vi "RT Driver VI.vi"(7 "Operation":T1, 11 "Device Reference in":T2 format="%.0x") -> (0 "Error Code":i32)   [LabVIEW 2021, in "Modbus Master Engine.lvlib"]
uses:
  Modbus Master Engine.lvlib
  <vilib>/NI VeriStand/Custom Device API/Custom Device Item Ref.ctl
  <vilib>/NI VeriStand/Custom Device API/Hardware Interface Driver VI Operation.ctl
  Shared/Device Info.ctl
  Shared/Write Mode.ctl
  Shared/Controls/Interface Type.ctl
  Shared/Controls/Data Model/TCP Settings.ctl
  Shared/Controls/Data Model/Serial Settings.ctl
  SubVIs/Bulk Data Access.ctl
  System Explorer/SubVIs/Modbus Type.ctl
  Shared/Controls/Data Model/Channel.ctl
  <vilib>/NI VeriStand/Custom Device API/Custom Device Channel Type.ctl
  Shared/Controls/Data Model/Mapping.ctl
  Shared/Controls/Data Model/DataType.ctl
  RTStateData.ctl
  <vilib>/NI/NIVS Inline Async API/_VS Inline Async API/VS Inline Async API/VS Inline Async API.lvclass
  <vilib>/NI/NIVS Inline Async API/_VS Inline Async API/VS Inline Async API/VS Inline Async API.lvclass/VS Inline Async API.ctl
  <vilib>/NI/NIVS Inline Async API/_Data Access Engine/Data Access Engine/Data Access Engine.lvclass/Data Access Engine.ctl
  <vilib>/NI/NIVS Inline Async API/_Data Access Engine/Access Type Classes/Write/Write.lvclass/Write.ctl
  <vilib>/NI/NIVS Inline Async API/_Data Access Engine/Access Type Classes/ReadWrite/ReadWrite.lvclass/ReadWrite.ctl
  <vilib>/NI/NIVS Inline Async API/_Data Access Engine/Access Type Classes/Read/Read.lvclass/Read.ctl
  <vilib>/NI/NIVS Inline Async API/_Data Access Engine/Data Access Engine/Methods/Data.Engine.Read Data from HW.vi
  <vilib>/NI/NIVS Inline Async API/_VS Inline Async API/Error Handling Process/SubVIs/Error.GetError.vi
  <vilib>/NI/NIVS Inline Async API/_Data Access Engine/Data Access Engine/Methods/Data.Engine.Write Data to HW.vi
  <vilib>/NI/NIVS Inline Async API/_Data Access Engine/Access Type Classes/ReadWrite/ReadWrite.EngineData.vi
  <vilib>/NI/NIVS Inline Async API/_Data Access Engine/Access Type Classes/Write/Write.EngineData.vi
  <vilib>/NI/NIVS Inline Async API/_Data Access Engine/Access Type Classes/Read/Read.EngineData.vi
  <vilib>/NI VeriStand/Custom Device API/NI VeriStand - Get Channel Value by Data Reference.vi
  <vilib>/NI VeriStand/Custom Device API/NI VeriStand - Set Channel Value by Data Reference.vi
  <vilib>/NI VeriStand/Custom Device API/NI VeriStand - Get Channel Values by Block Data Reference.vi
  Modbus Async.vi
  Shared/Constants.vi
  <vilib>/NI VeriStand/Custom Device API/Get Item Property (Variant).vi
  <vilib>/NI VeriStand/Custom Device API/Global Data Refs.vi
  <vilib>/NI VeriStand/Custom Device API/Custom Device API.lvlib
  Shared/Modbus Master Shared.lvlib
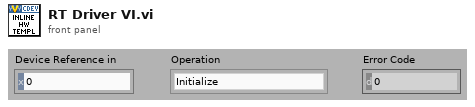
[diagram p1: front panel]
types:
  T1 = typedef "Custom Device API.lvlib/Hardware Interface Driver VI Operation.ctl" = enum16{"Initialize", "Start", "Read Data from HW", "Write Data to HW", "Close"}
  T2 = typedef "Custom Device API.lvlib/Custom Device Item Ref.ctl" = u64
  T3 = typedef "Modbus Master Engine.lvlib/RTStateData.ctl" = cluster{"Async":refnum<class "VS Inline Async API.lvclass">, "Device Info":T4}
  T4 = typedef "Modbus Master Shared.lvlib/Device Info.ctl" = cluster{"Interface Data":cluster{"Name":string, "Unit ID":u8, "Refresh Rate":i32, "Write Rate":i32, "Write Mode":T5, "Interface Type":T6, "TCP Settings":T7, "Serial Settings":T8}, "Modbus Input Groups":T9[], "Modbus Output Groups":T9[], "error in (no error)":errorcluster, "Modbus Input Engine Group Names":string[], "Modbus Output Engine Group Names":string[]}
  T5 = typedef "Modbus Master Shared.lvlib/Write Mode.ctl" = enum16{"Value Change", "Interval"}
  T6 = typedef "Modbus Master Shared.lvlib/Interface Type.ctl" = enum16{"TCP Master", "Serial Master", "TCP Slave", "Serial Slave"}
  T7 = typedef "Modbus Master Shared.lvlib/TCP Settings.ctl" = cluster{"Address":string, "Port":u16, "Timeout":i32}
  T8 = typedef "Modbus Master Shared.lvlib/Serial Settings.ctl" = cluster{"VISA resource name":refnum<visa-resource-name>, "baud rate":u32, "parity (even)":u16, "flow control (none)":u16, "serial type":enum16{"RTU", "ASCII"}, "Wire Mode":i16}
  T9 = typedef "Modbus Master Shared.lvlib/Bulk Data Access.ctl" = cluster{"Modbus Type":T10, "start":u16, "length":u16, "Channel Data":T11[]}
  T10 = typedef "Modbus Master Shared.lvlib/Modbus Type.ctl" = enum16{"Coil", "Discrete Input", "Holding Register", "Input Register"}
  T11 = typedef "Modbus Master Shared.lvlib/Channel.ctl" = cluster{"Name":string, "Modbus Type":T10, "Veristand Type":T12, "Mapping":T13}
  T12 = typedef "Custom Device API.lvlib/Custom Device Channel Type.ctl" = enum16{"Input", "Output"}
  T13 = typedef "Modbus Master Shared.lvlib/Mapping.ctl" = cluster{"DataType":T14, "Starting Address":u16, "Sub-Index (Bool)":u16, "VS Reference":T2}
  T14 = typedef "Modbus Master Shared.lvlib/DataType.ctl" = enum16{"Double", "Single", "I64", "I32", "I16", "I8", "U64", "U32", "U16", "U8", "Boolean"}
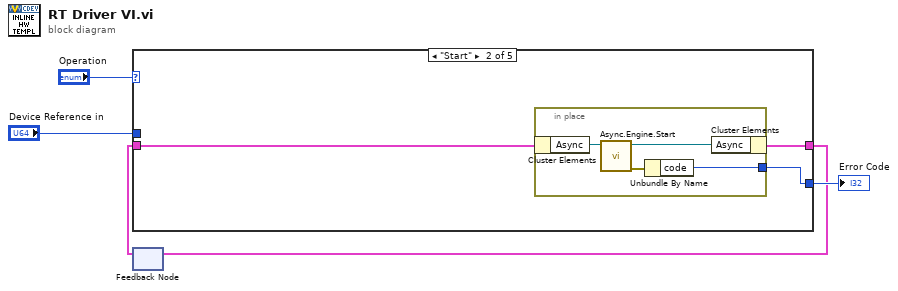
[diagram p0: block diagram]
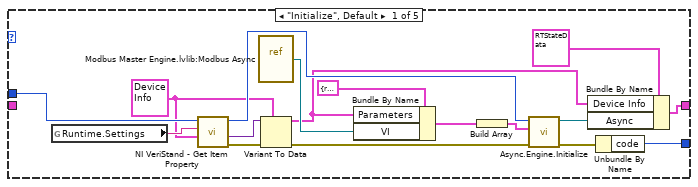
[diagram p2: hidden frame]
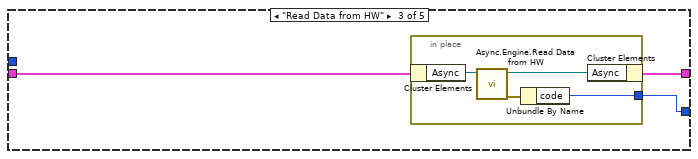
[diagram p3: hidden frame]
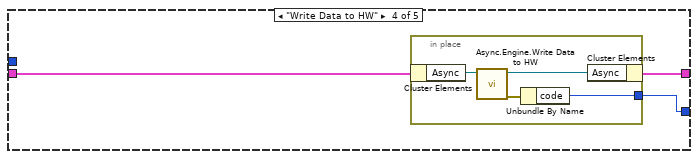
[diagram p4: hidden frame]
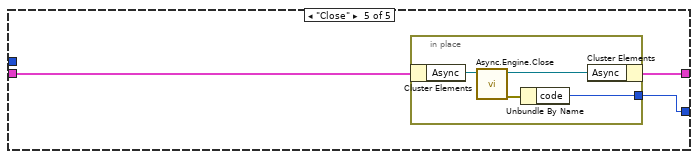
[diagram p5: hidden frame]
diagram:
  n1 = feedback #1() -> (w1:T3)  [unwired: 1 out]
  n2 = case shown="\"Start\"" "Operation" {
    tunnel: [w21 w24 w30 w37 w45] -> w2
    tunnel: w1 -> [_ w25 w32 w38 w46]
    tunnel: "Device Reference in" -> [w17 _ _ _ _]
    tunnel: [w22 w23 w31 w39 w44] -> w3
    frame "Initialize", Default {
      w13 = T4 {"Interface Data"={"Name"="", "Unit ID"=0, "Refresh Rate"=0, "Write Rate"=0, "Write Mode"=enum."Value Change", "Interface Type"=enum."TCP Master", "TCP Settings"={"Address"="", "Port"=2, "Timeout"=0}, "Serial Settings"={"VISA resource name"="", "baud rate"=0, "parity (even)"=0, "flow control (none)"=0, "serial type"=enum."RTU", "Wire Mode"=-1}}, "Modbus Input Groups"=[], "Modbus Output Groups"=[], "error in (no error)"={"status"=FALSE, "code"=0, "source"=""}, "Modbus Input Engine Group Names"=[], "Modbus Output Engine Group Names"=[]} ("Device Info")
      n3 = global read "Constants.vi" "Runtime.Settings"() -> (w14:string)
      n4 = call-poly <vilib>:"NI VeriStand - Get Item Property.vi"("Default Value"=w13, "Property Name"=w14, "Item Ref in"=w17) -> ("error out"=w7:errorcluster, "Value"=w16:variant, "Item Ref out"=w15:T2)  [unwired: 5 in, 1 out]
      n5 = vi-ref "Modbus Master Engine.lvlib:Modbus Async.vi"() -> (w19:refnum<vi>)
      n6 = Variant To Data(error in=w7, type=w13, Variant=w16) -> (data=w12:T4, error out=w8:errorcluster)
      n7 = Bundle By Name(cluster=cluster{"VI":refnum<vi>, "Parameters":variant} {"VI"=refnum, "Parameters"=variant} ("Process"), "Parameters"=w12, "VI"=w19) -> (w18:cluster{"VI":refnum<vi>, "Parameters":variant})
      n8 = Build Array(w18) -> (w10:cluster{"VI":refnum<vi>, "Parameters":variant}[])
      n9 = call <vilib>:"Async.Engine.Initialize.vi"("error in (no error)"=w8, "Processes"=w10, "Custom Device Ref"=w15) -> ("error out"=w6:errorcluster, "Async"=w11:refnum<class "VS Inline Async API.lvclass">)  [unwired: 7 in]
      n10 = Bundle By Name(cluster=T3 {"Async"=refnum, "Device Info"={"Interface Data"={"Name"="", "Unit ID"=0, "Refresh Rate"=0, "Write Rate"=0, "Write Mode"=enum."Value Change", "Interface Type"=enum."TCP Master", "TCP Settings"={"Address"="", "Port"=2, "Timeout"=0}, "Serial Settings"={"VISA resource name"="", "baud rate"=0, "parity (even)"=0, "flow control (none)"=0, "serial type"=enum."RTU", "Wire Mode"=-1}}, "Modbus Input Groups"=[], "Modbus Output Groups"=[], "error in (no error)"={"status"=FALSE, "code"=0, "source"=""}, "Modbus Input Engine Group Names"=[], "Modbus Output Engine Group Names"=[]}}, "Device Info"=w12, "Async"=w11) -> (w21:T3)
      n11 = Unbundle By Name(w6) -> ("code"=w22:i32)
    }
    frame "Start" {
      n12 = in-place {
        in-place-border: [w27] -> w23
        n13 = in-place-cluster #2(w25) -> ("Async"=w26:refnum<class "VS Inline Async API.lvclass">)
        n14 = call <vilib>:"Async.Engine.Start.vi"("VS Inline Async API in"=w26) -> ("error out"=w28:errorcluster, "VS Inline Async API out"=w29:refnum<class "VS Inline Async API.lvclass">)  [unwired: 9 in]
        n15 = Unbundle By Name(w28) -> ("code"=w27:i32)
        n16 = in-place-cluster #2("Async"=w29) -> (w24:T3)
      }
    }
    frame "Read Data from HW" {
      n17 = in-place {
        in-place-border: [w35] -> w31
        n18 = in-place-cluster #3(w32) -> ("Async"=w33:refnum<class "VS Inline Async API.lvclass">)
        n19 = call <vilib>:"Async.Engine.Read Data from HW.vi"("Async in"=w33) -> ("error out"=w34:errorcluster, "Async out"=w36:refnum<class "VS Inline Async API.lvclass">)  [unwired: 9 in]
        n20 = Unbundle By Name(w34) -> ("code"=w35:i32)
        n21 = in-place-cluster #3("Async"=w36) -> (w30:T3)
      }
    }
    frame "Write Data to HW" {
      n22 = in-place {
        in-place-border: [w43] -> w39
        n23 = in-place-cluster #4(w38) -> ("Async"=w40:refnum<class "VS Inline Async API.lvclass">)
        n24 = call <vilib>:"Async.Engine.Write Data to HW.vi"("VS Inline Async API in"=w40) -> ("error out"=w42:errorcluster, "VS Inline Async API out"=w41:refnum<class "VS Inline Async API.lvclass">)  [unwired: 9 in]
        n25 = Unbundle By Name(w42) -> ("code"=w43:i32)
        n26 = in-place-cluster #4("Async"=w41) -> (w37:T3)
      }
    }
    frame "Close" {
      n27 = in-place {
        in-place-border: [w49] -> w44
        n28 = in-place-cluster #5(w46) -> ("Async"=w47:refnum<class "VS Inline Async API.lvclass">)
        n29 = call <vilib>:"Async.Engine.Close.vi"("Async in"=w47) -> ("error out"=w48:errorcluster, "Async out"=w50:refnum<class "VS Inline Async API.lvclass">)  [unwired: 9 in]
        n30 = Unbundle By Name(w48) -> ("code"=w49:i32)
        n31 = in-place-cluster #5("Async"=w50) -> (w45:T3)
      }
    }
  }
  "Error Code" <- w3
  n32 = feedback-in #1(w2) -> ()
